vi "Read Requests.vi"(11 "JQMHModule in":refnum<class "Module.lvclass">) -> (2 "Requests":T1, 3 "JQMHModule out":refnum<class "Module.lvclass">)   [LabVIEW 2024, in "Module.lvclass"]
uses:
  Module.lvclass
  Module.lvclass/Module.ctl
  StopEventArgs.ctl
  StandardRequests.ctl
  Show Front Panel--Args.ctl
  Hide Front Panel.ctl
  Show Block Diagram.ctl
  Hide Block Diagram--Args.ctl
  Reply.ctl
  InitialiseArgs.ctl
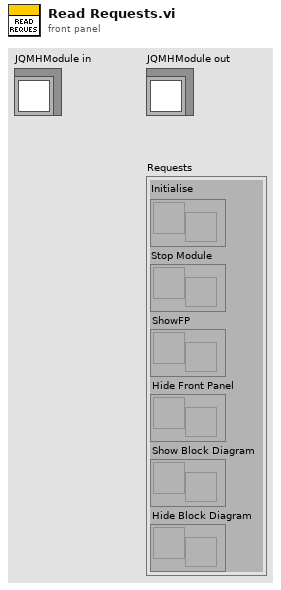
[diagram p1: front panel]
types:
  T1 = typedef "Module.lvclass/StandardRequests.ctl" = cluster{"Initialise":refnum<user-event>, "Stop Module":refnum<user-event>, "ShowFP":refnum<user-event>, "Hide Front Panel":refnum<user-event>, "Show Block Diagram":refnum<user-event>, "Hide Block Diagram":refnum<user-event>}
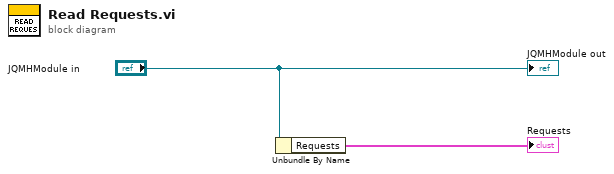
[diagram p0: block diagram]
diagram:
  n1 = Unbundle By Name("JQMHModule in") -> ("Requests"=→"Requests":T1)
  "JQMHModule out" <- "JQMHModule in"
